vi "Fault Handling.vi"(8 "error in (no error)":errorcluster, 10 "FaultCode":i32, 11 "PreUUT in":refnum<class "PreUUT.lvclass">) -> (0 "error out":errorcluster, 2 "Fault codes":cluster{"Bit":string, "Description":string}[](array[cluster]), 3 "PreUUT out":refnum<class "PreUUT.lvclass">)   [LabVIEW 2021, in "OPC UA.lvlib" / "PreUUT.lvclass"]
uses:
  PreUUT.lvclass
  PreUUT.lvclass/PreUUT.ctl
  OPC UA/OPC UA.lvclass
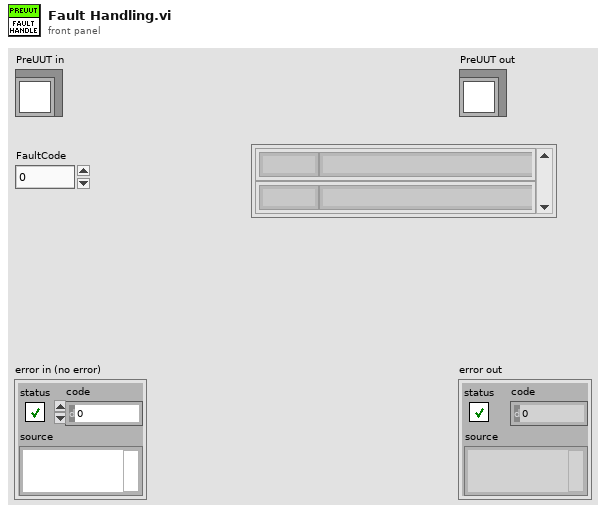
[diagram p1: front panel]
types:
  T1 = typedef "PreUUT.lvclass/Rx PreUUT.ctl" = cluster{"NestStatus":bool, "PalletID":u32, "Start":bool, "BarcodeData":string, "FaultCode":u32, "Stop":bool}
  T2 = typedef "PreUUT.lvclass/Tx PreUUT.ctl" = cluster{"Online":bool, "Ready":bool, "Fault":bool, "Timeout":bool, "Results":u32, "StepNo":u32, "TestRunning":bool, "ResultsReady":bool}
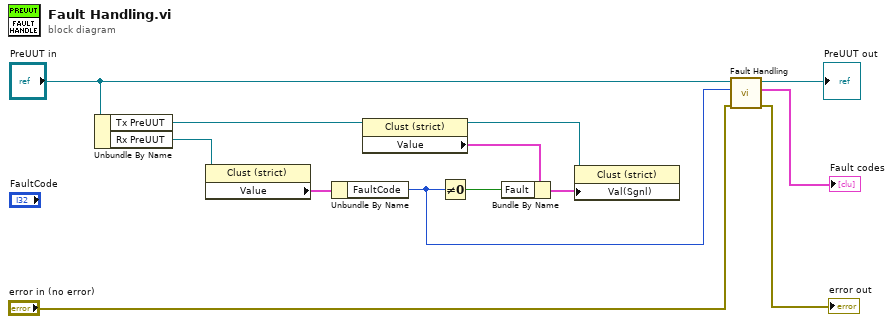
[diagram p0: block diagram]
diagram:
  n1 = Unbundle By Name("PreUUT in") -> ("Tx PreUUT"=w9:refnum<vi>, "Rx PreUUT"=w12:refnum<vi>)
  n2 = property class="Clust (strict)"(reference=w12) -> ("Value"=w11:T1)  [unwired: 1 in, 2 out]
  n3 = Unbundle By Name(w11) -> ("FaultCode"=w4:u32)
  n4 = property class="Clust (strict)"(reference=w9) -> (reference out=w7:refnum<vi>, "Value"=w5:T2)  [unwired: 1 in, 1 out]
  n5 = Not Equal To 0?(x=w4) -> (x != 0?=w2:bool)
  n6 = Bundle By Name(cluster=w5, "Fault"=w2) -> (w8:T2)
  n7 = property class="Clust (strict)"(reference=w7, "Val(Sgnl)"=w8) -> ()  [unwired: 1 in, 2 out]
  n8 = call-parent "Fault Handling.vi"("error in (no error)"="error in (no error)", "FaultCode"=w4, "OPC UA in"="PreUUT in") -> ("error out"=→"error out":errorcluster, "Fault codes"=→"Fault codes":cluster{"Bit":string, "Description":string}[], "OPC UA out"=→"PreUUT out":refnum<class "PreUUT.lvclass">)  [unwired: 6 in]
